vi "ICNC Ramp Up Abs Buf.vi"(0 "Axis":u32, 1 "FInc":u32[](array[numeric])=[0, 0, 0, 0, 0], 5 "Position":i32[](array[numeric])=[0, 0, 0, 0, 0], 7 "FStart":u32[](array[numeric])=[0, 0, 0, 0, 0], 9 "FEnd":u32[](array[numeric])=[0, 0, 0, 0, 0], 11 "error in (no error)":errorcluster caption="entrée d'erreur (pas d'erreur)") -> (3 "FInc out":u32[](array[numeric]), 4 "function return":u32, 6 "Position out":i32[](array[numeric]), 8 "FStart out":u32[](array[numeric]), 10 "FEnd out":u32[](array[numeric]), 15 "error out":errorcluster caption="sortie d'erreur")   [LabVIEW 2012, in "ICNC2.lvlib"]
doc: "DWORD ICNC_RampUpAbsBuf( DWORD Axis,\n INT Position[5],\n DWORD FStart[5],\n DWORD FEnd[5],\n DWORD FInc[5]);"
uses:
  <userlib>/ICNC/ICNC2.lvlib
  <userlib>/ICNC/ICNC2.dll
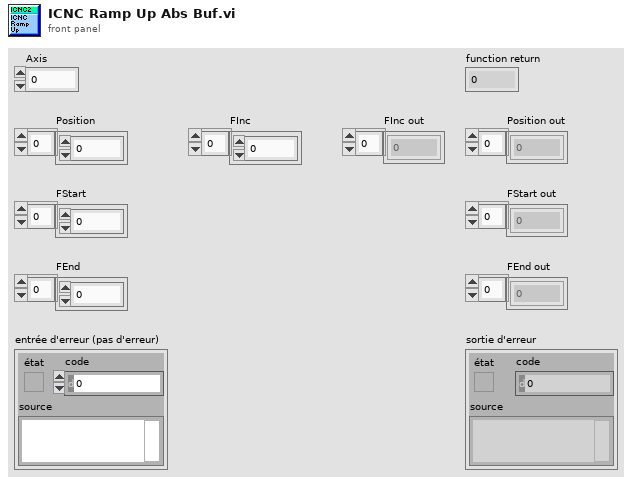
[diagram p1: front panel]
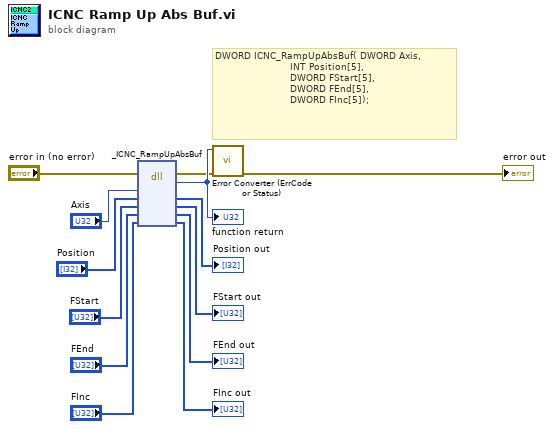
[diagram p0: block diagram]
diagram:
  # "DWORD ICNC_RampUpAbsBuf( DWORD Axis,\n                         INT Position[5],\n                         DWORD FStart[5],\n                         DWORD FEnd[5],\n                         DWORD FInc[5]);"
  n1 = dll-call lib="C:/Program Files (x86)/National Instruments/LabVIEW 2012/user.lib/ICNC/ICNC2.*" fn="_ICNC_RampUpAbsBuf"(error in="error in (no error)", "Axis"="Axis", "Position"="Position", "FStart"="FStart", "FEnd"="FEnd", "FInc"="FInc") -> (error out=w2:errorcluster, w13:u32, "Position"=→"Position out":i32[], "FStart"=→"FStart out":u32[], "FEnd"=→"FEnd out":u32[], "FInc"=→"FInc out":u32[])  [unwired: 3 in, 1 out]
  "function return" <- w13
  n2 = call <userlib>:"Error Converter (ErrCode or Status).vi"("error in (no error)"=w2, "error code"=w13) -> ("error out"=→"error out":errorcluster)  [unwired: 9 in]
